vi "Post-Install.vi"(10 "Variant":variant) -> (0 "error out":errorcluster)   [LabVIEW 2024]
uses:
  <vilib>/regexp/Match Regular Expression.xnode
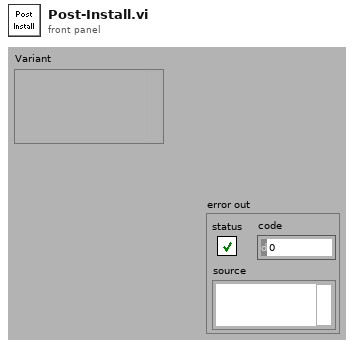
[diagram p1: front panel]
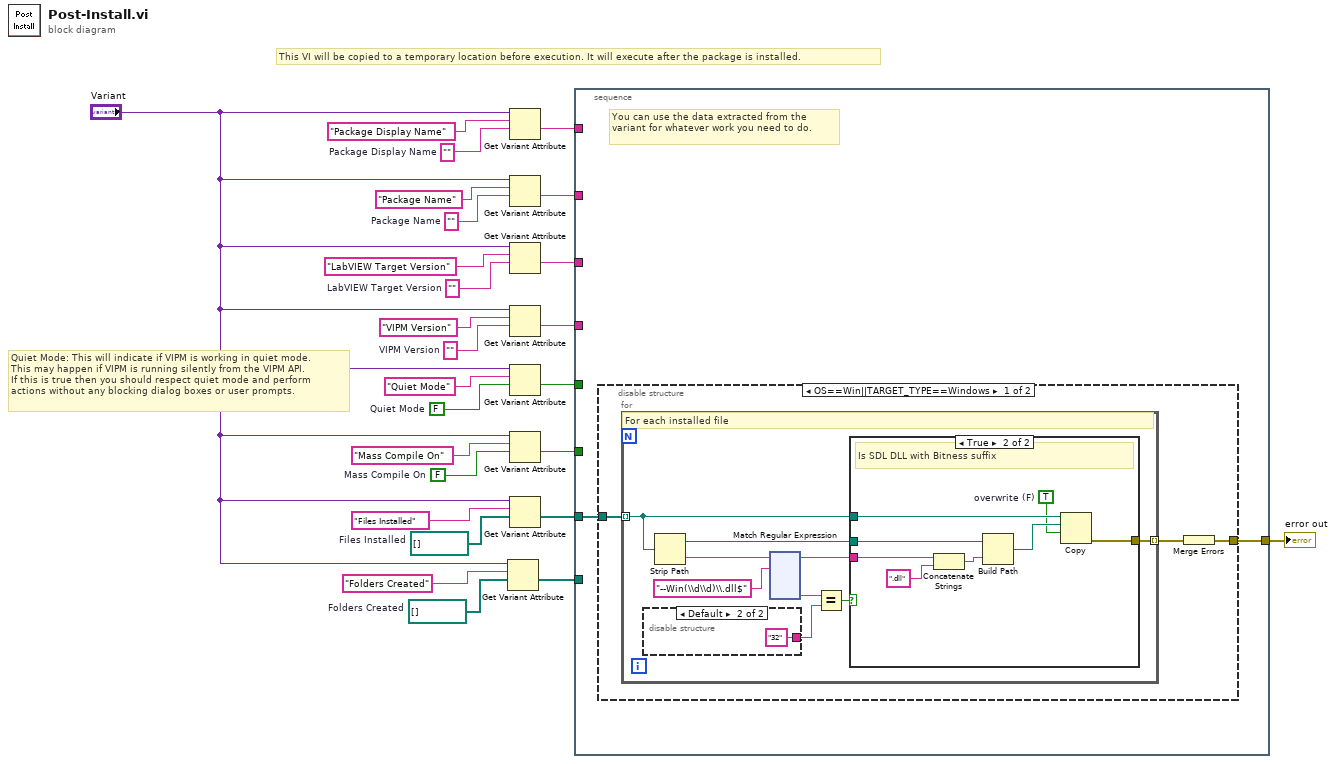
[diagram p0: block diagram]
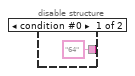
[diagram p2: hidden frame]
diagram:
  w2 = path[] []  # Folders Created
  w3 = path[] []  # Files Installed
  w9 = FALSE  # Mass Compile On
  w10 = ""  # Package Display Name
  w17 = FALSE  # Quiet Mode
  w20 = ""  # VIPM Version
  w22 = ""  # LabVIEW Target Version
  w24 = ""  # Package Name
  # "Quiet Mode: This will indicate if VIPM is working in quiet mode.\nThis may happen if VIPM is running silently from the VIPM API.\nIf this is true then you should respect quiet mode and perform\nactions without any blocking dialog boxes or user prompts."
  # "This VI will be copied to a temporary location before execution. It will execute after the package is installed."
  n1 = Get Variant Attribute(Variant="Variant", name="Folders Created", default value (empty Variant)=w2) -> (value=w7:path[])  [unwired: 1 in, 3 out]
  n2 = Get Variant Attribute(Variant="Variant", name="Package Display Name", default value (empty Variant)=w10) -> (value=w16:string)  [unwired: 1 in, 3 out]
  n3 = Get Variant Attribute(Variant="Variant", name="Package Name", default value (empty Variant)=w24) -> (value=w15:string)  [unwired: 1 in, 3 out]
  n4 = Get Variant Attribute(Variant="Variant", name="LabVIEW Target Version", default value (empty Variant)=w22) -> (value=w14:string)  [unwired: 1 in, 3 out]
  n5 = Get Variant Attribute(Variant="Variant", name="VIPM Version", default value (empty Variant)=w20) -> (value=w13:string)  [unwired: 1 in, 3 out]
  n6 = Get Variant Attribute(Variant="Variant", name="Quiet Mode", default value (empty Variant)=w17) -> (value=w12:bool)  [unwired: 1 in, 3 out]
  n7 = Get Variant Attribute(Variant="Variant", name="Mass Compile On", default value (empty Variant)=w9) -> (value=w11:bool)  [unwired: 1 in, 3 out]
  n8 = Get Variant Attribute(Variant="Variant", name="Files Installed", default value (empty Variant)=w3) -> (value=w6:path[])  [unwired: 1 in, 3 out]
  n9 = stacked-sequence {
    tunnel: w16 -> [_]
    tunnel: w15 -> [_]
    tunnel: w14 -> [_]
    tunnel: w13 -> [_]
    tunnel: w12 -> [_]
    tunnel: w11 -> [_]
    tunnel: w6 -> [w28]
    tunnel: w7 -> [_]
    tunnel: [w27] -> w1
    frame #0 {
      # "You can use the data extracted from the variant for whatever work you need to do."
      n10 = disable-structure shown="OS==Win||TARGET_TYPE==Windows" {
        disable-tunnel: w28 -> [w31 _]
        disable-tunnel: [w29 _] -> w27
        frame condition #0 (active) {
          n11 = for {
            tunnel: w31 -> [w33] mode=indexing
            tunnel: [w32] -> w30 mode=indexing
            # "For each installed file"
            n12 = disable-structure shown="Default" {
              disable-tunnel: ["64" "32"] -> w37
              frame condition #0 {
              }
              frame condition #1 (active) {
              }
            }
            n13 = Strip Path(path=w33) -> (stripped path=w34:path, name=w40:string)
            n14 = xnode "Match Regular Expression"("input string"=w40, "regular expression"="--Win(\\d\\d)\\.dll$") -> ("before match"=w35:string, "submatch 1"=w38:string)  [unwired: 4 in, 4 out]
            n15 = Equal?(x=w38, y=w37) -> (x = y?=w36:bool)
            n16 = case shown="True" w36 {
              tunnel: w35 -> [_ w49]
              tunnel: w34 -> [_ w50]
              tunnel: w33 -> [_ w46]
              tunnel: [_ w43] -> w32
              frame False {
                # "Do nothing"
                # "Not SDL DLL with Bitness suffix"
              }
              frame True {
                w44 = TRUE  # overwrite (F)
                # "Is SDL DLL with Bitness suffix"
                n17 = Concatenate Strings(w49, ".dll" ("string")) -> (w48:string)
                n18 = Build Path(base path=w50, name or relative path=w48) -> (appended path=w45:path)
                n19 = Copy(9:w44, 10:w45, 11:w46) -> (0:w43:errorcluster)  [unwired: 2 in, 2 out]
              }
            }
          }
          n20 = Merge Errors(w30) -> (w29:errorcluster)
        }
        frame condition #1 {
          # "Do nothing for linux"
        }
      }
    }
  }
  "error out" <- w1
